vi "Shutdown.vi"(8 "error in":errorcluster, 11 "RDMA Transceiver in":refnum<class "RDMA Transceiver.lvclass">) -> (0 "error out":errorcluster, 3 "RDMA Transceiver out":refnum<class "RDMA Transceiver.lvclass">)   [LabVIEW 2020, in "RDMA.lvlib" / "RDMA Transceiver.lvclass"]
doc: "Executes when the deployment is terminated (regardless of error state) and closes all RDMA sessions."
uses:
  RDMA Transceiver.lvclass
  RDMA Transceiver.lvclass/RDMA Transceiver.ctl
  Transfer Group Parameters.ctl
  Transfer Parameters.ctl
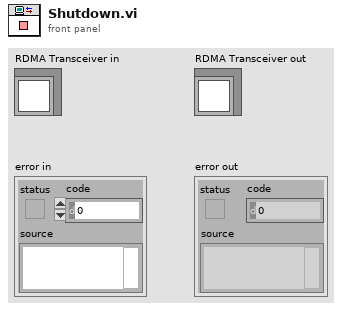
[diagram p1: front panel]
types:
  T1 = typedef "RDMA.lvlib/RDMA Transceiver.lvclass/Transfer Group Parameters.ctl" = cluster{"transfers":T2[]}
  T2 = typedef "RDMA.lvlib/RDMA Transceiver.lvclass/Transfer Parameters.ctl" = cluster{"connected session":refnum<k21>, "listener session":refnum<k21>}
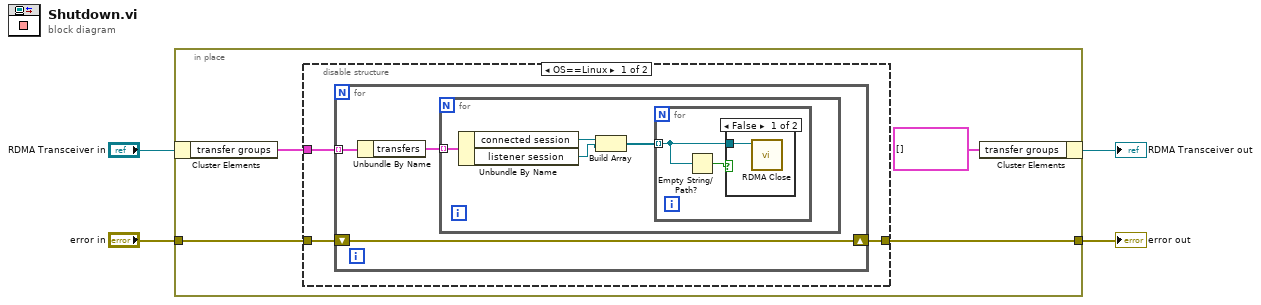
[diagram p0: block diagram]
diagram:
  n1 = in-place {
    in-place-border: "error in" -> [w5]
    in-place-border: [w7] -> w1
    n2 = in-place-cluster #1("RDMA Transceiver in") -> ("transfer groups"=w6:T1[])
    n3 = disable-structure shown="OS==Linux" {
      disable-tunnel: w5 -> [w11 w22]
      disable-tunnel: [w10 w22] -> w7
      disable-tunnel: w6 -> [w9 _]
      frame condition #0 (active) {
        n4 = for {
          shift-right: [w12] -> w10
          shift-left: w11 -> [w12]
          tunnel: w9 -> [w14] mode=indexing
          n5 = Unbundle By Name(w14) -> ("transfers"=w13:T2[])
          n6 = for {
            tunnel: w13 -> [w18] mode=indexing
            n7 = Unbundle By Name(w18) -> ("connected session"=w17:refnum<k21>, "listener session"=w16:refnum<k21>)
            n8 = Build Array(w17, w16) -> (w15:refnum<k21>[])
            n9 = for {
              tunnel: w15 -> [w20] mode=indexing
              n10 = Empty String/Path?(string/path=w20) -> (empty?=w19:bool)
              n11 = case shown="False" w19 {
                tunnel: w20 -> [w21 _]
                frame False {
                  n12 = call <vilib>:"RDMA Close.vi"("rdma session"=w21) -> ()  [unwired: 10 in, 1 out]
                }
                frame True {
                }
              }
            }
          }
        }
      }
      frame condition #1 {
      }
    }
    n13 = in-place-cluster #1("transfer groups"=T1[] [] ("Transfer Group parameters")) -> (→"RDMA Transceiver out":refnum<class "RDMA Transceiver.lvclass">)
  }
  "error out" <- w1
